vi "Read Calibration File.vi"(0 "Filepath":path=path "C:/Rolls Royce/JackScrew.cal") -> (1 "NumPages":i32, 2 "TotalLines":i32, 3 "CalData":T1(array[cluster]) {"ChlFactor" format="%.3f"; "ChlZero" format="%.3f"}, 4 "PageTitles":string[](array[string]), 6 "ErrOut":bool)   [LabVIEW 2013]
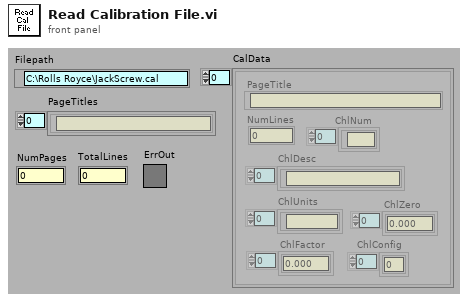
[diagram p1: front panel]
types:
  T1 = cluster{"PageTitle":string, "NumLines":i32, "ChlNum":string[], "ChlDesc":string[], "ChlUnits":string[], "ChlZero":sgl[], "ChlFactor":sgl[], "ChlConfig":u16[]}[]
  T2 = cluster{"PageTitle":string, "NumLines":i32, "ChlNum":string[], "ChlDesc":string[], "ChlUnits":string[], "ChlZero":sgl[], "ChlFactor":sgl[], "ChlConfig":u16[]}
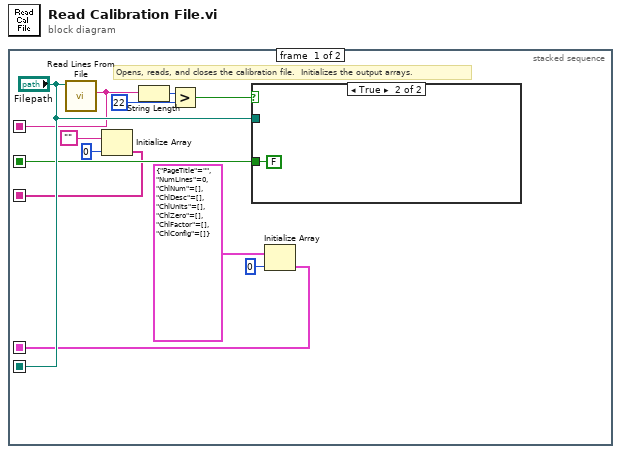
[diagram p0: block diagram]
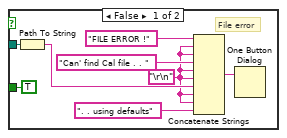
[diagram p2: hidden frame]
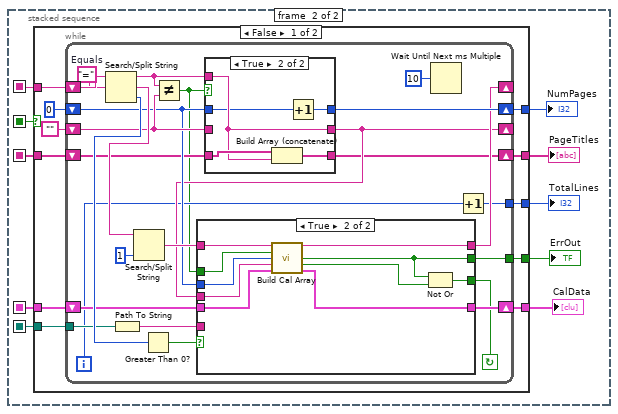
[diagram p3: hidden frame]
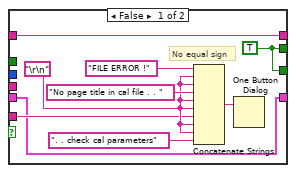
[diagram p5: hidden frame]
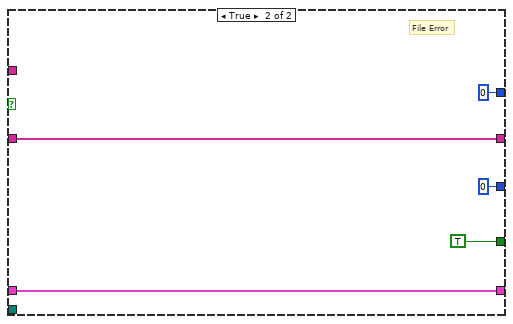
[diagram p6: hidden frame]
diagram:
  n1 = stacked-sequence {
    seq-local: [w9 _] -> [_ w30]
    seq-local: [w8 _] -> [_ w31]
    seq-local: ["Filepath" _] -> [_ w29]
    seq-local: [w6 _] -> [_ w27]
    seq-local: [w2 _] -> [_ w25]
    frame #0 {
      # "Opens, reads, and closes the calibration file.  Initializes the output arrays."
      n2 = call <vilib>:"Read Lines From File.vi"("file path (dialog if empty)"="Filepath") -> ("line string"=w9:string)  [unwired: 5 in, 3 out]
      n3 = Initialize Array("", 0 ("Dimension Size")) -> (w2:string[])
      n4 = String Length(string=w9) -> (length=w11:i32)
      n5 = Greater?(x=w11, y=22) -> (0:w5:bool)
      n6 = case shown="True" w5 {
        tunnel: "Filepath" -> [w14 _]
        tunnel: [TRUE FALSE] -> w8
        frame False {
          w16 = "\r\n"
          # "File error"
          n7 = Path To String(path=w14) -> (string=w17:string)
          n8 = Concatenate Strings("FILE ERROR !", w16, w16, "Can' find Cal file . . ", w16, w16, w17, w16, w16, ". . using defaults") -> (w19:string)
          n9 = One Button Dialog(message=w19) -> ()  [unwired: 1 in, 1 out]
        }
        frame True {
        }
      }
      n10 = Initialize Array(T2 {"PageTitle"="", "NumLines"=0, "ChlNum"=[], "ChlDesc"=[], "ChlUnits"=[], "ChlZero"=[], "ChlFactor"=[], "ChlConfig"=[]} ("Output Array"), 0 ("Dimension Size")) -> (w6:T1)
    }
    frame #1 {
      n11 = case shown="False" w31 {
        tunnel: w30 -> [w42 _]
        tunnel: w29 -> [w41 _]
        tunnel: [w38 0] -> w28
        tunnel: w27 -> [w37 w98]
        tunnel: [w36 w98] -> w26
        tunnel: w25 -> [w35 w97]
        tunnel: [w34 w97] -> w24
        tunnel: [w33 TRUE ("Err")] -> w23
        tunnel: [w32 0] -> w22
        frame False {
          n12 = while {
            tunnel: [w46] -> w32
            tunnel: [w48] -> w33
            shift-left: w35 -> [w50]
            shift-right: [w49] -> w34
            shift-left: w37 -> [w52]
            shift-right: [w51] -> w36
            shift-left: 0 -> [w54]
            shift-right: [w60] -> w38
            shift-left: "" -> [w58]
            shift-right: [w53] -> _
            tunnel: w41 -> [w62]
            shift-left: w42 -> [w65]
            shift-right: [w55] -> _
            i -> [w45]
            stop <- w47 continue-if-true
            w64 = "="  # Equals
            n13 = Search/Split String(string=w65, search string/char (-)=w64) -> (substring before match=w59:string, match + rest of string=w67:string, offset of match=w63:i32)  [unwired: 1 in]
            n14 = Path To String(path=w62) -> (string=w61:string)
            n15 = Search/Split String(string=w67, offset (0)=1) -> (match + rest of string=w56:string)  [unwired: 1 in, 2 out]
            n16 = Greater Than 0?(x=w63) -> (x > 0?=w57:bool)
            n17 = Not Equal?(x=w59, y=w58) -> (x != y?=w43:bool)
            n18 = case shown="True" w43 {
              tunnel: [w70 w75] -> w60
              tunnel: [w69 w72] -> w53
              tunnel: w54 -> [w70 w71]
              tunnel: w59 -> [_ w72]
              tunnel: w58 -> [w69 _]
              tunnel: w50 -> [w68 w73]
              tunnel: [w68 w74] -> w49
              frame False {
              }
              frame True {
                n19 = Build Array (concatenate)(w73, w72) -> (w74:string[])
                n20 = Increment(x=w71) -> (x+1=w75:i32)
              }
            }
            n21 = case shown="True" w57 {
              tunnel: w61 -> [w79 _]
              tunnel: w56 -> [w78 w94]
              tunnel: [w78 w93] -> w55
              tunnel: w43 -> [_ w92]
              tunnel: w54 -> [_ w91]
              tunnel: w53 -> [_ w90]
              tunnel: w52 -> [w77 w89]
              tunnel: [w77 w88] -> w51
              tunnel: [w76 w86] -> w48
              tunnel: [w76 w87] -> w47
              frame False {
                w76 = TRUE ("Err")
                w81 = "\r\n"
                # "No equal sign"
                n22 = Concatenate Strings("FILE ERROR !", w81, w81, "No page title in cal file . . ", w81, w81, w79, w81, w81, ". . check cal parameters") -> (w83:string)
                n23 = One Button Dialog(message=w83) -> ()  [unwired: 1 in, 1 out]
              }
              frame True {
                n24 = call "Build Cal Array.vi"("TextIn"=w94, "NewPage"=w92, "PageNum"=w91, "PageTitle"=w90, "CalDataIn"=w89) -> ("TextOut"=w93:string, "Err"=w86:bool, "Done"=w85:bool, "CalDataOut"=w88:T1)  [unwired: 7 in]
                n25 = Not Or(1:w85, 2:w86) -> (0:w87:bool)
              }
            }
            n26 = Wait Until Next ms Multiple(millisecond multiple=u32 10) -> ()  [unwired: 1 out]
            n27 = Increment(x=w45) -> (x+1=w46:i32)
          }
        }
        frame True {
          # "File Error"
        }
      }
      "ErrOut" <- w23
      "CalData" <- w26
      "PageTitles" <- w24
      "TotalLines" <- w22
      "NumPages" <- w28
    }
  }
